vi "Control Digital IO Pin.vi"(8 "error in (no error)":errorcluster, 9 "Pin Value":bool, 10 "Pin Index":u8) -> (0 "error out":errorcluster, 1 "Pin Value Out":bool, 2 "Pin Index Out":u8)   [LabVIEW 2020, in "FirmataClient.lvlib"]
doc: "Allows requesting the state of a digital pin."
uses:
  FirmataClient.lvlib
  Controls/FirmataPinModes.ctl
  Transports/Controls/Transport Commands.ctl
panel:
  in  "Queue Name":string="firmata-serial-communication"
  out "Pin Mode":T1=enum."Extended.DHT"
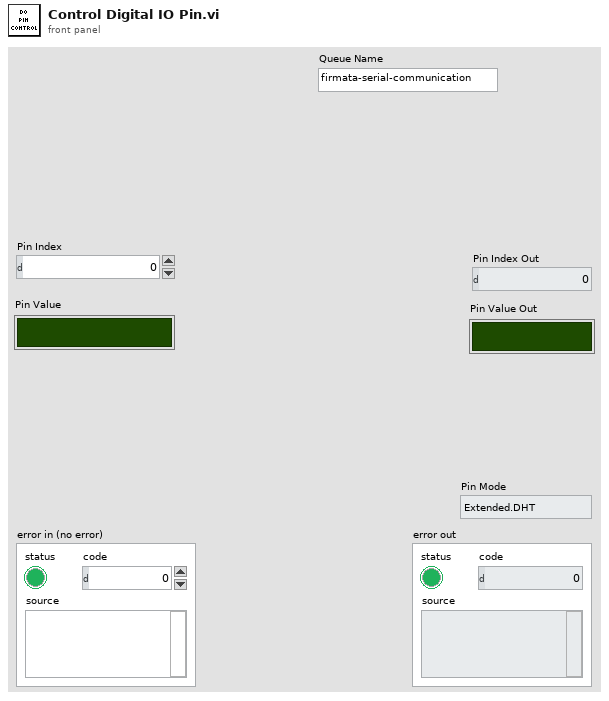
[diagram p1: front panel]
types:
  T1 = typedef "FirmataClient.lvlib/FirmataPinModes.ctl" = enum16{"DigitalInput", "DigitalOutput", "AnalogInput", "PWM", "Servo", "Shift", "I2C", "OneWire", "Stepper", "Encoder", "Serial", "InputPullup", "Extended.SPI", "Extended.Sonar", "Extended.Tone", "Extended.DHT"}
  T2 = typedef "Transport Commands.ctl" = enum16{"Initialize", "Transmit - Receive", "Cleanup", "Cleanup And Stop"}
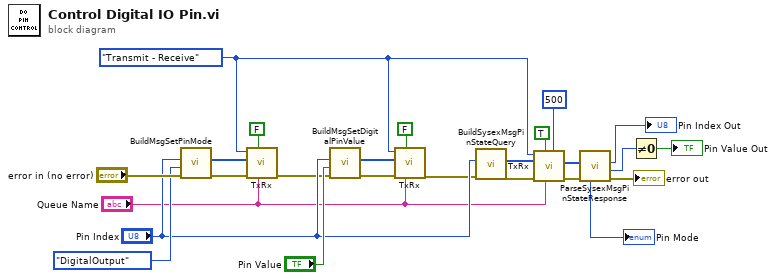
[diagram p0: block diagram]
diagram:
  w1 = Transport_Commands."Transmit - Receive" ("Command")
  n1 = call "BuildMsgSetPinMode.vi"("error in"="error in (no error)", "Pin Mode"=FirmataPinModes."DigitalOutput", "Pin Index"="Pin Index") -> ("error out"=w15:errorcluster, "SetPinModeMessage"=w14:u8[])  [unwired: 5 in, 2 out]
  n2 = call "TxRx.vi"("Queue Name"="Queue Name", "Wait For Reply?"=FALSE, "error in"=w15, "Message"=w14, "Command"=w1) -> ("error out"=w10:errorcluster)  [unwired: 5 in, 1 out]
  n3 = call "BuildMsgSetDigitalPinValue.vi"("error in"=w10, "Pin Value"="Pin Value", "Pin Index"="Pin Index") -> ("error out"=w12:errorcluster, "DigitalPinValueMessage"=w11:u8[])  [unwired: 5 in, 2 out]
  n4 = call "TxRx.vi"("Queue Name"="Queue Name", "Wait For Reply?"=FALSE, "error in"=w12, "Message"=w11, "Command"=w1) -> ("error out"=w5:errorcluster)  [unwired: 5 in, 1 out]
  n5 = call "BuildSysexMsgPinStateQuery.vi"("error in"=w5, "Pin Index"="Pin Index") -> ("error out"=w6:errorcluster, "GetPinStateMessage"=w7:u8[])  [unwired: 6 in, 2 out]
  n6 = call "TxRx.vi"("Reply Timeout Ms"=500, "Queue Name"="Queue Name", "Wait For Reply?"=TRUE, "error in"=w6, "Message"=w7, "Command"=w1) -> ("error out"=w4:errorcluster, "Reply"=w3:u8[])  [unwired: 4 in]
  n7 = call "ParseSysexMsgPinStateResponse.vi"("error in"=w4, "Sysex Message"=w3) -> ("error out"=→"error out":errorcluster, "Pin State"=w18:u64, "Pin Index"=→"Pin Index Out":u8, "Pin Mode"=→"Pin Mode":T1)  [unwired: 6 in]
  n8 = Not Equal To 0?(x=w18) -> (x != 0?=→"Pin Value Out":bool)
